vi "AlazarGetDriverVersion.vi"(11 "error in (no error)":errorcluster) -> (4 "Major Number":u8, 6 "Minor Number":u8, 8 "Revision Number":u8, 10 "Return Code":u32, 15 "error out":errorcluster)   [LabVIEW 2009]
doc: "Get the device driver version of the most recently opened device."
uses:
  ATSApi.dll
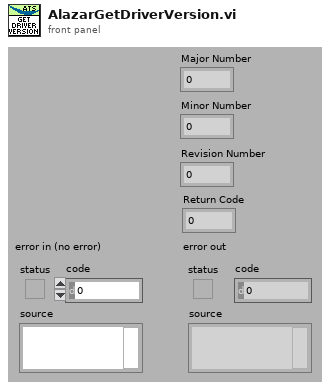
[diagram p1: front panel]
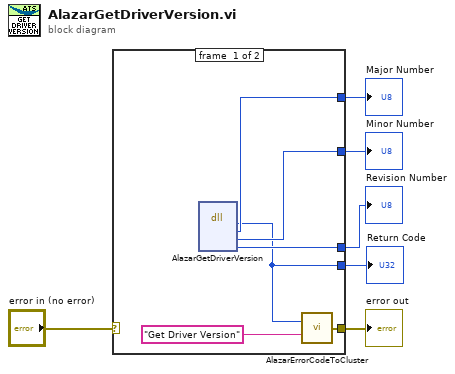
[diagram p0: block diagram]
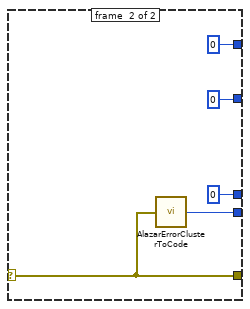
[diagram p2: hidden frame]
diagram:
  n1 = case shown="No Error" "error in (no error)" {
    selector: "error in (no error)" -> [_ w17]
    tunnel: [w9 w17] -> w5
    tunnel: [w8 w16] -> w4
    tunnel: [w12 0] -> w3
    tunnel: [w11 0] -> w2
    tunnel: [w10 0] -> w1
    frame #0 {
      n2 = dll-call lib="ATSApi.dll" fn="AlazarGetDriverVersion"() -> (w8:u32, "majorNumber"=w12:u8, "minorNumber"=w11:u8, "revisionNumber"=w10:u8)  [unwired: 6 in, 2 out]
      n3 = call "AlazarErrorCodeToCluster.vi"("Message"="Get Driver Version", "Error Code"=w8) -> ("error out"=w9:errorcluster)
    }
    frame #1 {
      n4 = call "AlazarErrorClusterToCode.vi"("error in (no error)"=w17) -> ("Error Code"=w16:u32)
    }
  }
  "error out" <- w5
  "Return Code" <- w4
  "Revision Number" <- w1
  "Minor Number" <- w2
  "Major Number" <- w3
